vi "Write Test Type.vi"(7 "Command":string="init", 11 "Test":string="init") -> (3 "Test":string)   [LabVIEW 2014]
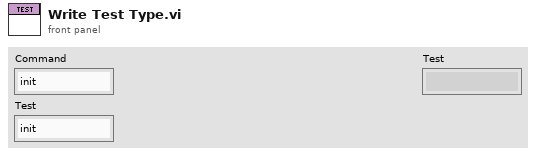
[diagram p1: front panel]
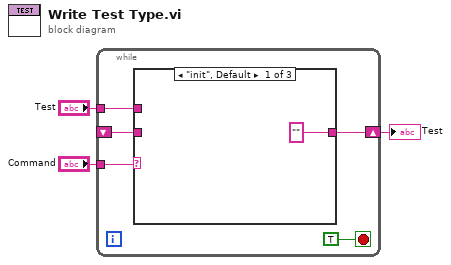
[diagram p0: block diagram]
diagram:
  n1 = while {
    tunnel: "Command" -> [w7]
    shift-right: [w5] -> w1
    shift-left: _ -> [w6]
    tunnel: "Test" -> [w4]
    stop <- TRUE stop-if-true
    n2 = case shown="\"init\", Default" w7 {
      tunnel: w6 -> [_ _ w11]
      tunnel: ["" w10 w11] -> w5
      tunnel: w4 -> [_ w10 _]
      frame "init", Default {
      }
      frame "write" {
      }
      frame "read" {
      }
    }
  }
  "Test" <- w1
